vi "Convert_StringToDBL.vi"(9 "node text":string) -> (1 "Numeric":dbl format="%.2f")   [LabVIEW 2010, in "Pansino_XML_Read.lvlib"]
uses:
  Pansino_XML_Read.lvlib
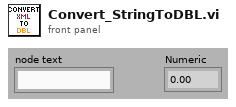
[diagram p1: front panel]
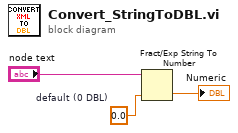
[diagram p0: block diagram]
diagram:
  w2 = 0.0  # default (0 DBL)
  n1 = Fract/Exp String To Number(string="node text", default (0 dbl)=w2) -> (number=→"Numeric":dbl)  [unwired: 2 in, 1 out]
